vi "GRG Create Arbitrary Waveform.vi"(6 "Timeout (10000)":i32=10000, 8 "error in (no error)":errorcluster, 10 "Arbitrary Waveform Name (\"ARB1\")":string="ARB1", 11 "VISA resource name":refnum<visa-resource-name>) -> (0 "error out":errorcluster, 3 "VISA resource name out":refnum<visa-resource-name>)   [LabVIEW 2011]
doc: "Creates and saves an arbitrary (user-defined) waveform in non-volatile memory. \n\n<B>Note:</B>\n \n(1) Data is scaled and normalized so that the waveform will be centered around y=0. Models 33120A and 33250A have 12-bit digitizers and will be scaled from -2047 to +2047. Model 33210A and 33220A has a 14-bit digitizer and will be scaled from -8191 to + 8191.\n\n(2) Call Configure Arbitrary Waveform VI to set the arbitrary waveform as the active function.\n\n(3) Creates an arbitrary waveform in non-volatile memory and because of this, the waveform will remain stored on the instrument until deleted. If any sensitive information is contained in the arbitrary waveform, it is recommended that the waveform be deleted when finished"
uses:
  <instrlib>/Agilent 33XXX Series/Agilent 33XXX Series.lvlib
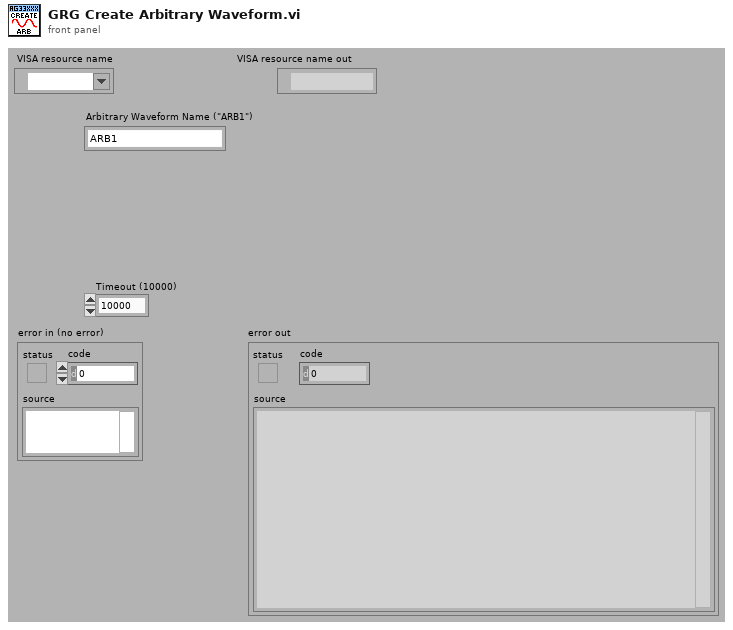
[diagram p1: front panel]
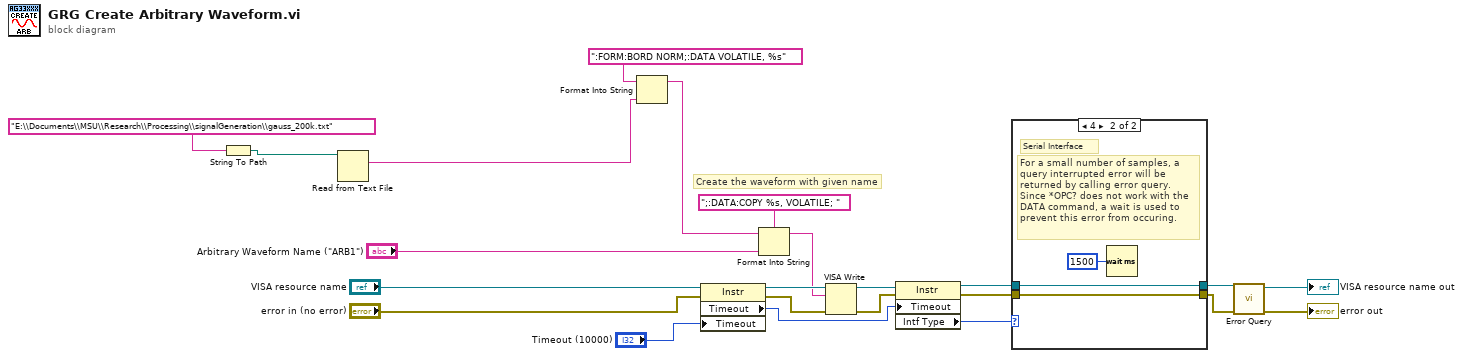
[diagram p0: block diagram]
diagram:
  # "Create the waveform with given name"
  n1 = String To Path(string="E:\\Documents\\MSU\\Research\\Processing\\signalGeneration\\gauss_200k.txt") -> (path=w2:path)
  n2 = Read from Text File(file (use dialog)=w2) -> (text=w1:string)  [unwired: 3 in, 3 out]
  n3 = Format Into String(format string=":FORM:BORD NORM;:DATA VOLATILE, %s" ("string"), w1) -> (resulting string=w15:string)  [unwired: 2 in, 1 out]
  n4 = property on="Property Node" class="Instr"(reference="VISA resource name", error in="error in (no error)", "Timeout"="Timeout (10000)") -> (reference out=w22:refnum<visa-resource-name>, error out=w23:errorcluster, "Timeout"=w19:u32)
  n5 = Format Into String(format string=";:DATA:COPY %s, VOLATILE; ", initial string=w15, "Arbitrary Waveform Name (\"ARB1\")") -> (resulting string=w13:string)  [unwired: 1 in, 1 out]
  n6 = VISA Write(VISA resource name=w22, write buffer=w13, error in (no error)=w23) -> (VISA resource name out=w21:refnum<visa-resource-name>, error out=w20:errorcluster)  [unwired: 1 out]
  n7 = property on="Property Node" class="Instr"(reference=w21, error in=w20, "Timeout"=w19) -> (reference out=w12:refnum<visa-resource-name>, error out=w10:errorcluster, "Intf Type"=w8:u16)
  n8 = case shown="4" w8 {
    tunnel: w12 -> [w25 w28]
    tunnel: [w25 w28] -> w11
    tunnel: w10 -> [w24 w27]
    tunnel: [w24 w27] -> w9
    frame 0, Default {
    }
    frame 4 {
      # "For a small number of samples, a query interrupted error will be returned by calling error query.  Since *OPC? does not work with the DATA command, a wait is used to prevent this error from occuring."
      # "Serial Interface"
      n9 = Wait (ms)(milliseconds to wait=u32 1500) -> ()  [unwired: 1 out]
    }
  }
  n10 = call <instrlib>:"Error Query.vi"("error in (no error)"=w9, "VISA resource name"=w11) -> ("error out"=→"error out":errorcluster, "VISA resource name out"=→"VISA resource name out":refnum<visa-resource-name>)  [unwired: 6 in, 2 out]
